vi "DisplayPanel.vi"() -> ()   [LabVIEW 2011]
uses:
  MvLVLib/MvCameraControl.lvlib
  MvLVLib/VIs/CreateGigEHandle.vi
  MvLVLib/VIs/CreateU3VHandle.vi
  <vilib>/picture/picture.llb/imagedata.ctl
panel:
  out "U3VDeviceArray":T1(array[cluster])
  out "GigEDeviceArray":T2(array[cluster])
  in  "pConvertInfo In":T3
  out "PixelFormat":u32
  out "handle out":u64
  in  "handle":u64
  in  "Rectangle":T4
  in  "image data":T5 caption="图像数据"
  out "Picture":picture
  out "PayloadSize":u32
  out "pFrameInfoEx out":T6
  out "nHeight":u32
  out "nWidth":u32
  out "Acquisision Flag":bool
  in  "Trigger Mode":bool
  in  "Continuous":bool
  out "打开标志":bool
  in  "stop":bool
  in  "Trigger Once":bool
  in  "Stop":bool
  in  "Start":bool
  in  "Open Device":bool
  in  "Close Device":bool
  in  "error in (no error) 2":errorcluster caption="错误输入（无错误）"
  in  "Refresh Devices":bool
  in  "Device List":u16(ring)
  # "Initialize"
  # "Acquisition"
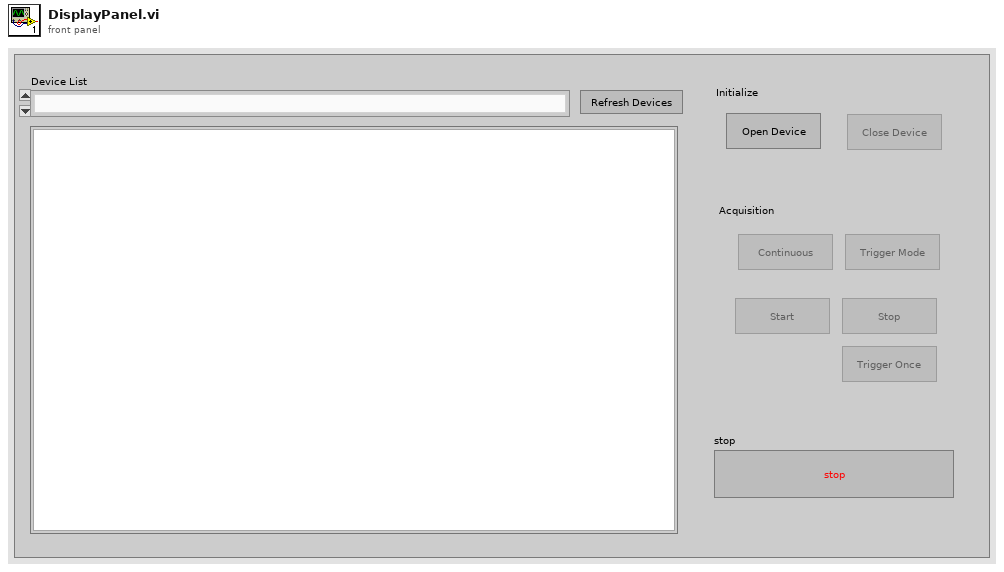
[diagram p1: front panel]
types:
  T1 = cluster{"nMajorVer":u16, "nMinorVer":u16, "nMacAddrHigh":u32, "nMacAddrLow":u32, "nTLayerType":u32, "nReserved0":u32, "nReserved1":u32, "nReserved2":u32, "nReserved3":u32, "CrtlInEndPoint":u8, "CrtlOutEndPoint":u8, "StreamEndPoint":u8, "EventEndPoint":u8, "idVendor":u16, "idProduct":u16, "nDeviceNumber":u32, "nRes0":u32, "nRes1":u32, "chDeviceGUID":string, "chVendorName":string, "chModelName":string, "chFamilyName":string, "chDeviceVersion":string, "chManufacturerName":string, "chSerialNumber":string, "chUserDefinedName":string, "nbcdUSB":u32, "nRes2":u32, "nRes3":u32}[]
  T2 = cluster{"nMajorVer":u16, "nMinorVer":u16, "nMacAddrHigh":u32, "nMacAddrLow":u32, "nTLayerType":u32, "nReserved0":u32, "nReserved1":u32, "nReserved2":u32, "nReserved3":u32, "nIpCfgOption":u32, "nIpCfgCurrent":u32, "nCurrentIp":u32, "nCurrentSubNetMask":u32, "nDefaultGateWay":u32, "chManualfacturerName":string, "chModelName":string, "chDeviceVersion":string, "chManufacturerSpecificInfo":string, "chSerialNumber":string, "chUserDefinedName":string, "nRes0":string, "nRes1":string, "nNetExport":u32, "nRes2":u32, "nRes3":u32}[]
  T3 = cluster{"nWidth":u16, "nHeight":u16, "enSrcPixelType":u32, "nSrcDataLen":u32, "enDstPixelType":u32, "nDstLen":u32, "nDstBufferSize":u32, "nRes0":u32, "nRes1":u32, "nRes2":u32, "nRes3":u32}
  T4 = cluster{"left":i16, "top":i16, "right":i16, "bottom":i16}
  T5 = typedef "imagedata.ctl" = cluster{"image type":i32, "image depth":i32, "image":u8[], "mask":u8[], "colors":u32[], "Rectangle":cluster{"left":i16, "top":i16, "right":i16, "bottom":i16}}
  T6 = cluster{"nWidth":u16, "nHeight":u16, "enPixelType":i32, "nFrameNum":u32, "nDevTimeStampHigh":u32, "nDevTimeStampLow":u32, "nReserved0":u32, "nHostTimeStamp":i64, "nFrameLen":u32, "nSecondCount]":u32, "nCycleCount":u32, "nCycleOffset":u32, "fGain":u32, "fExposureTime":u32, "nAverageBrightness":u32, "nRed":u32, "nGreen":u32, "nBlue":u32, "nFrameCounter":u32, "nTriggerIndex":u32, "nInput":u32, "nOutput":u32, "nOffsetX":u32, "nOffsetY":u32, "nReserved[0]":u32, "nReserved[1]":u32, "nReserved[2]":u32, "nReserved[3]":u32, "nReserved[4]":u32, "nReserved[5]":u32, "nReserved[6]":u32, "nReserved[7]":u32, "nReserved[8]":u32, "nReserved[9]":u32, "nReserved[10]":u32, "nReserved[11]":u32, "nReserved[12]":u32, "nReserved[13]":u32, "nReserved[14] 10":u32, "nReserved[15] 11":u32, "nReserved[16] 12":u32, "nReserved[17] 13":u32, "nReserved[18] 14":u32, "nReserved[19] 15":u32, "nReserved[20] 16":u32, "nReserved[21] 17":u32, "nReserved[22] 18":u32, "nReserved[23] 19":u32, "nReserved[24] 20":u32, "nReserved[25] 21":u32, "nReserved[26] 22":u32, "nReserved[27] 23":u32, "nReserved[28] 24":u32, "nReserved[29] 25":u32, "nReserved[30] 26":u32, "nReserved[31] 27":u32, "nReserved[32] 28":u32, "nReserved[33] 29":u32, "nReserved[34] 30":u32, "nReserved[35] 31":u32, "nReserved[36] 32":u32, "nReserved[37] 33":u32, "nReserved[38] 34":u32, "nReserved[39] 35":u32, "nReserved[40] 36":u32}
  T7 = enum8{"Enabled", "Disabled", "Disabled and Grayed Out"}
  T8 = cluster{"nCurValue":u32, "nMax":u32, "nMin":u32, "nInc":u32, "nReserved[0]":u32, "nReserved[1]":u32, "nReserved[2]":u32, "nReserved[3]":u32}
  T9 = cluster{"nCurValue":u32, "nSupportedNum":u32, "nSupportValue[0]":u32, "nSupportValue[1]":u32, "nSupportValue[2]":u32, "nSupportValue[3]":u32, "nSupportValue[4]":u32, "nSupportValue[5]":u32, "nSupportValue[6]":u32, "nSupportValue[7]":u32, "nSupportValue[8]":u32, "nSupportValue[9]":u32, "nSupportValue[10]":u32, "nSupportValue[11]":u32, "nSupportValue[12]":u32, "nSupportValue[13]":u32, "nSupportValue[14]":u32, "nSupportValue[15]":u32, "nSupportValue[16]":u32, "nSupportValue[17]":u32, "nSupportValue[18]":u32, "nSupportValue[19]":u32, "nSupportValue[20]":u32, "nSupportValue[21]":u32, "nSupportValue[22]":u32, "nSupportValue[23]":u32, "nSupportValue[24]":u32, "nSupportValue[25]":u32, "nSupportValue[26]":u32, "nSupportValue[27]":u32, "nSupportValue[28]":u32, "nSupportValue[29]":u32, "nSupportValue[30]":u32, "nSupportValue[31]":u32, "nSupportValue[32]":u32, "nSupportValue[33]":u32, "nSupportValue[34]":u32, "nSupportValue[35]":u32, "nSupportValue[36]":u32, "nSupportValue[37]":u32, "nSupportValue[38]":u32, "nSupportValue[39]":u32, "nSupportValue[40]":u32, "nSupportValue[41]":u32, "nSupportValue[42]":u32, "nSupportValue[43]":u32, "nSupportValue[44]":u32, "nSupportValue[45]":u32, "nSupportValue[46]":u32, "nSupportValue[47]":u32, "nSupportValue[48]":u32, "nSupportValue[49]":u32, "nSupportValue[50]":u32, "nSupportValue[51]":u32, "nSupportValue[52]":u32, "nSupportValue[53]":u32, "nSupportValue[54]":u32, "nSupportValue[55]":u32, "nSupportValue[56]":u32, "nSupportValue[57]":u32, "nSupportValue[58]":u32, "nSupportValue[59]":u32, "nSupportValue[60]":u32, "nSupportValue[61]":u32, "nSupportValue[62]":u32, "nSupportValue[63]":u32, "nReserved[0]":u32, "nReserved[1]":u32, "nReserved[2]":u32, "nReserved[3]":u32}
  T10 = cluster{"nMajorVer":u16, "nMinorVer":u16, "nMacAddrHigh":u32, "nMacAddrLow":u32, "nTLayerType":u32, "nReserved0":u32, "nReserved1":u32, "nReserved2":u32, "nReserved3":u32, "CrtlInEndPoint":u8, "CrtlOutEndPoint":u8, "StreamEndPoint":u8, "EventEndPoint":u8, "idVendor":u16, "idProduct":u16, "nDeviceNumber":u32, "nRes0":u32, "nRes1":u32, "chDeviceGUID":string, "chVendorName":string, "chModelName":string, "chFamilyName":string, "chDeviceVersion":string, "chManufacturerName":string, "chSerialNumber":string, "chUserDefinedName":string, "nbcdUSB":u32, "nRes2":u32, "nRes3":u32}
  T11 = cluster{"nMajorVer":u16, "nMinorVer":u16, "nMacAddrHigh":u32, "nMacAddrLow":u32, "nTLayerType":u32, "nReserved0":u32, "nReserved1":u32, "nReserved2":u32, "nReserved3":u32, "nIpCfgOption":u32, "nIpCfgCurrent":u32, "nCurrentIp":u32, "nCurrentSubNetMask":u32, "nDefaultGateWay":u32, "chManualfacturerName":string, "chModelName":string, "chDeviceVersion":string, "chManufacturerSpecificInfo":string, "chSerialNumber":string, "chUserDefinedName":string, "nRes0":string, "nRes1":string, "nNetExport":u32, "nRes2":u32, "nRes3":u32}
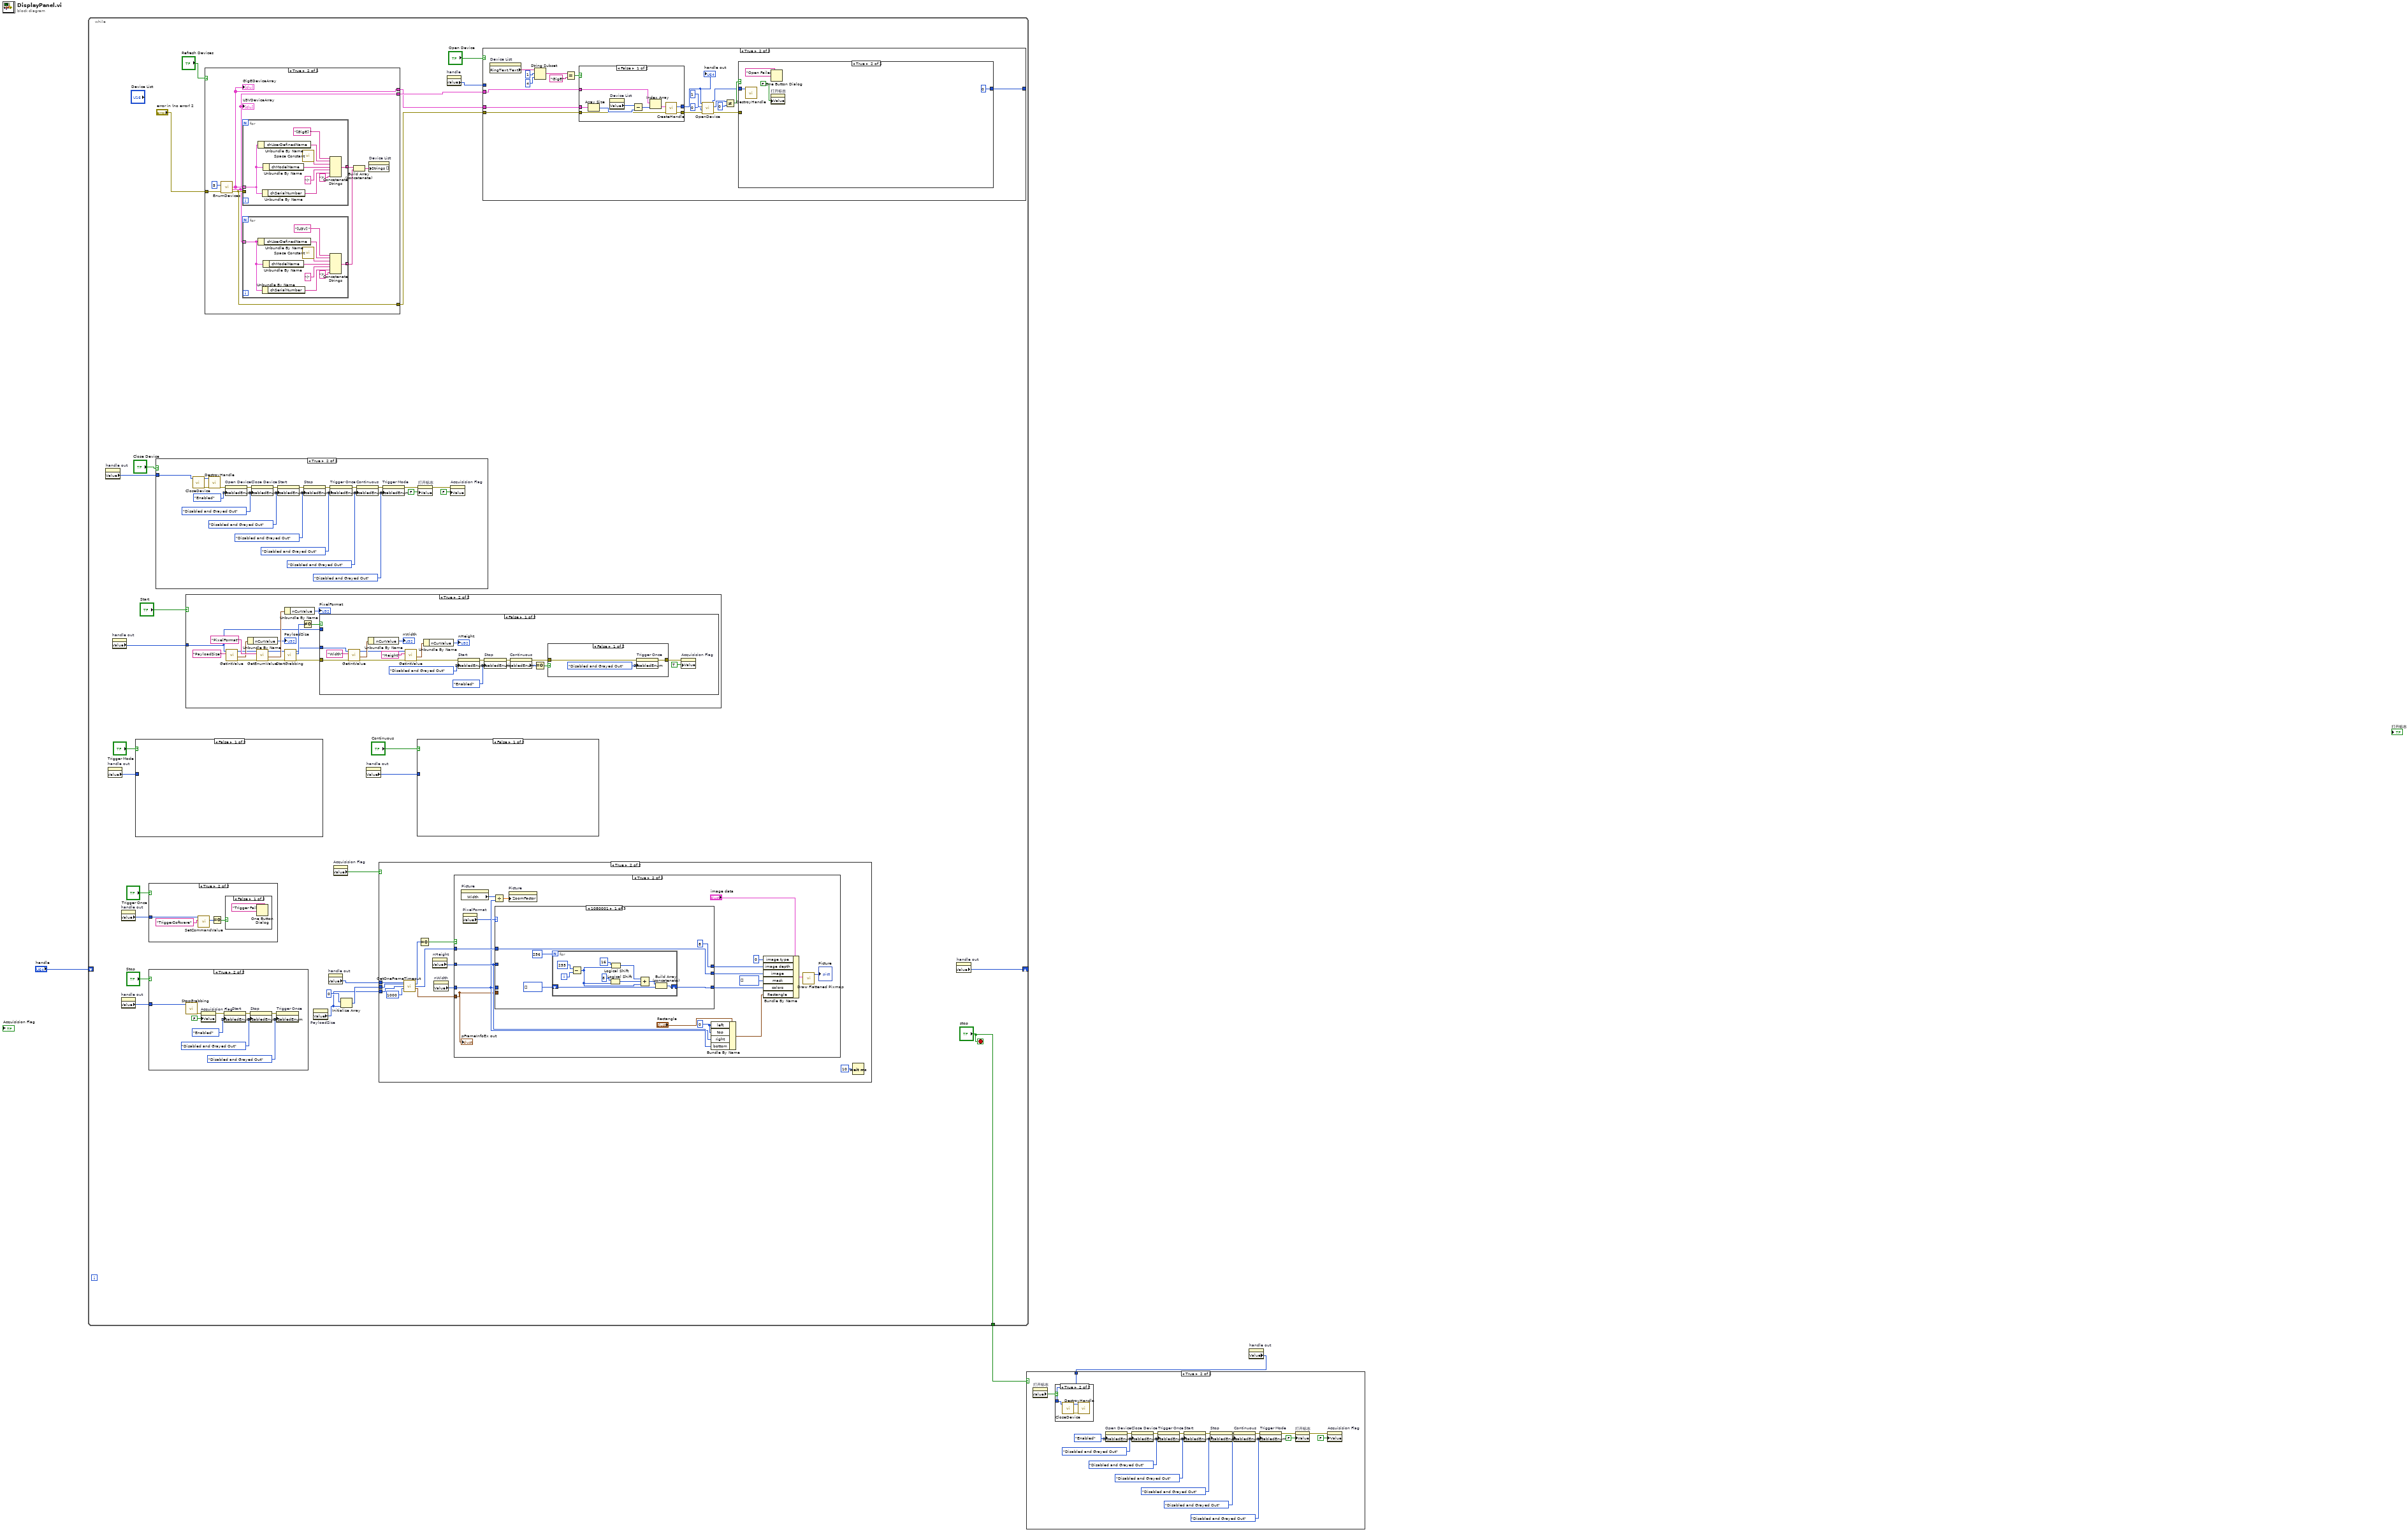
[diagram p0: block diagram]
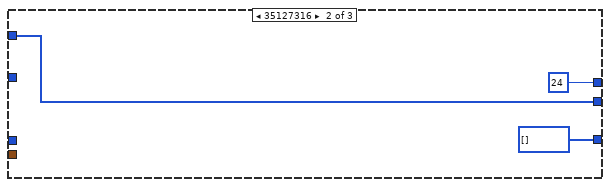
[diagram p6: hidden frame]
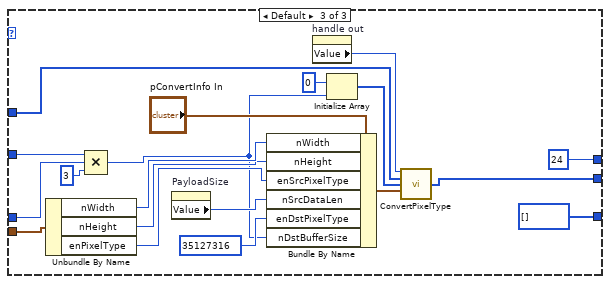
[diagram p7: hidden frame]
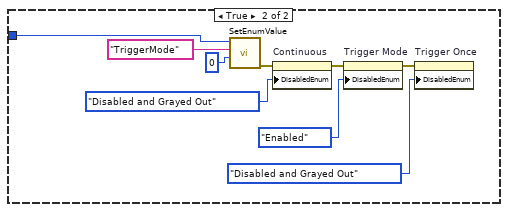
[diagram p9: hidden frame]
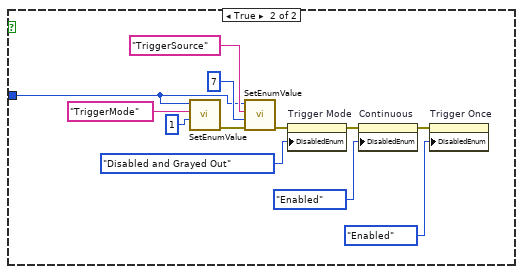
[diagram p10: hidden frame]
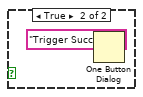
[diagram p12: hidden frame]
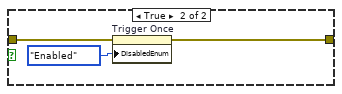
[diagram p14: hidden frame]
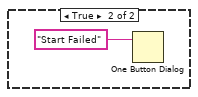
[diagram p15: hidden frame]
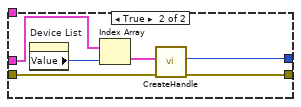
[diagram p18: hidden frame]
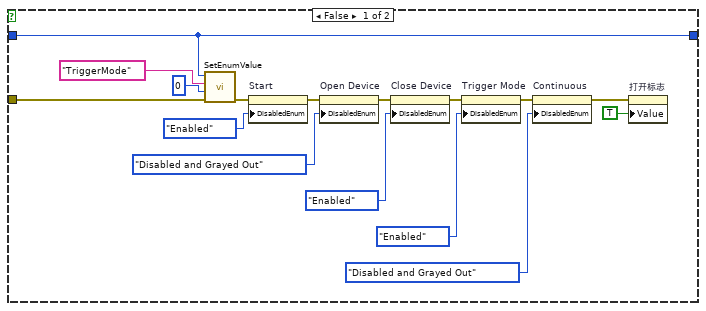
[diagram p19: hidden frame]
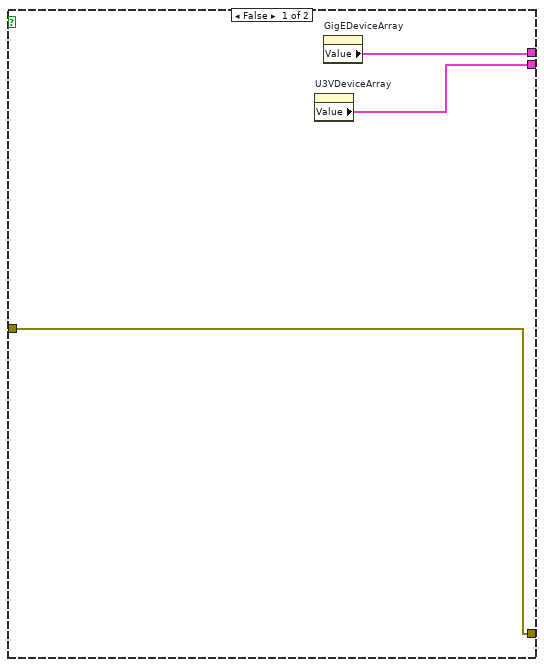
[diagram p20: hidden frame]
diagram:
  n1 = while {
    tunnel: ["stop"] -> w3
    shift-right: [w17] -> _
    shift-left: "handle" -> [_]
    stop <- "stop" stop-if-true
    n2 = property on="handle out" class="DigNum (strict)"() -> ("Value"=w15:u64)  [unwired: 2 in, 2 out]
    n3 = property on="handle out" class="DigNum (strict)"() -> ("Value"=w10:u64)  [unwired: 2 in, 2 out]
    n4 = property on="handle out" class="DigNum (strict)"() -> ("Value"=w11:u64)  [unwired: 2 in, 2 out]
    n5 = property on="handle out" class="DigNum (strict)"() -> ("Value"=w14:u64)  [unwired: 2 in, 2 out]
    n6 = property on="handle out" class="DigNum (strict)"() -> ("Value"=w13:u64)  [unwired: 2 in, 2 out]
    n7 = case shown="False" "Trigger Mode" {
      tunnel: w10 -> [_ w114]
      frame False {
      }
      frame True {
        n8 = call "SetEnumValue.vi"("nValue"=u32 1, "strKey"="TriggerMode", "handle"=w114) -> ("error out"=w120:errorcluster)  [unwired: 6 in, 2 out]
        n9 = call "SetEnumValue.vi"("error in (no error)"=w120, "nValue"=u32 7, "strKey"="TriggerSource", "handle"=w114) -> ("error out"=w119:errorcluster)  [unwired: 5 in, 2 out]
        n10 = property on="Trigger Mode" class="Bool"(error in=w119, "DisabledEnum"=T7."Disabled and Grayed Out" ("禁用")) -> (error out=w118:errorcluster)  [unwired: 1 in, 1 out]
        n11 = property on="Continuous" class="Bool"(error in=w118, "DisabledEnum"=T7."Enabled" ("禁用")) -> (error out=w116:errorcluster)  [unwired: 1 in, 1 out]
        n12 = property on="Trigger Once" class="Bool"(error in=w116, "DisabledEnum"=T7."Enabled" ("禁用")) -> ()  [unwired: 1 in, 2 out]
      }
    }
    n13 = case shown="True" "Trigger Once" {
      tunnel: w14 -> [_ w129]
      frame False {
      }
      frame True {
        n14 = call "SetCommandValue.vi"("strValue"="TriggerSoftware", "handle"=w129) -> ("function return"=w127:i32)  [unwired: 7 in, 2 out]
        n15 = Equal To 0?(x=w127) -> (x = 0?=w126:bool)
        n16 = case shown="False" w126 {
          frame False {
            n17 = One Button Dialog(message="Trigger Failed") -> ()  [unwired: 1 in, 1 out]
          }
          frame True {
            n18 = One Button Dialog(message="Trigger Success") -> ()  [unwired: 1 in, 1 out]
          }
        }
      }
    }
    n19 = case shown="True" "Stop" {
      tunnel: w13 -> [_ w104]
      frame False {
      }
      frame True {
        n20 = call "StopGrabbing.vi"("handle"=w104) -> ("error out"=w103:errorcluster)  [unwired: 8 in, 2 out]
        n21 = property on="Acquisision Flag" class="Bool (strict)"(error in=w103, "Value"=FALSE ("采集标志")) -> (error out=w98:errorcluster)  [unwired: 1 in, 1 out]
        n22 = property on="Start" class="Bool"(error in=w98, "DisabledEnum"=T7."Enabled" ("禁用")) -> (error out=w97:errorcluster)  [unwired: 1 in, 1 out]
        n23 = property on="Stop" class="Bool"(error in=w97, "DisabledEnum"=T7."Disabled and Grayed Out" ("禁用")) -> (error out=w96:errorcluster)  [unwired: 1 in, 1 out]
        n24 = property on="Trigger Once" class="Bool"(error in=w96, "DisabledEnum"=T7."Disabled and Grayed Out" ("禁用")) -> ()  [unwired: 1 in, 2 out]
      }
    }
    n25 = case shown="True" "Close Device" {
      tunnel: w15 -> [_ w175]
      frame False {
      }
      frame True {
        n26 = call "CloseDevice.vi"("handle"=w175) -> ("error out"=w177:errorcluster, "handle out"=w174:u64)  [unwired: 8 in, 1 out]
        n27 = call "DestroyHandle.vi"("error in (no error)"=w177, "handle"=w174) -> ("error out"=w176:errorcluster)  [unwired: 8 in, 1 out]
        n28 = property on="Open Device" class="Bool"(error in=w176, "DisabledEnum"=T7."Enabled" ("禁用")) -> (error out=w190:errorcluster)  [unwired: 1 in, 1 out]
        n29 = property on="Close Device" class="Bool"(error in=w190, "DisabledEnum"=T7."Disabled and Grayed Out" ("禁用")) -> (error out=w189:errorcluster)  [unwired: 1 in, 1 out]
        n30 = property on="Start" class="Bool"(error in=w189, "DisabledEnum"=T7."Disabled and Grayed Out" ("禁用")) -> (error out=w188:errorcluster)  [unwired: 1 in, 1 out]
        n31 = property on="Stop" class="Bool"(error in=w188, "DisabledEnum"=T7."Disabled and Grayed Out" ("禁用")) -> (error out=w187:errorcluster)  [unwired: 1 in, 1 out]
        n32 = property on="Trigger Once" class="Bool"(error in=w187, "DisabledEnum"=T7."Disabled and Grayed Out" ("禁用")) -> (error out=w184:errorcluster)  [unwired: 1 in, 1 out]
        n33 = property on="Continuous" class="Bool"(error in=w184, "DisabledEnum"=T7."Disabled and Grayed Out" ("禁用")) -> (error out=w182:errorcluster)  [unwired: 1 in, 1 out]
        n34 = property on="Trigger Mode" class="Bool"(error in=w182, "DisabledEnum"=T7."Disabled and Grayed Out" ("禁用")) -> (error out=w181:errorcluster)  [unwired: 1 in, 1 out]
        n35 = property on="打开标志" class="Bool (strict)"(error in=w181, "Value"=FALSE ("打开标志")) -> (error out=w179:errorcluster)  [unwired: 1 in, 1 out]
        n36 = property on="Acquisision Flag" class="Bool (strict)"(error in=w179, "Value"=FALSE ("采集标志")) -> ()  [unwired: 1 in, 2 out]
      }
    }
    n37 = case shown="True" "Start" {
      tunnel: w11 -> [_ w136]
      frame False {
      }
      frame True {
        n38 = call "GetIntValue.vi"("strKey"="PayloadSize", "handle"=w136) -> ("error out"=w142:errorcluster, "pIntValue out"=w138:T8, "handle out"=w134:u64)  [unwired: 6 in, 1 out]
        n39 = Unbundle By Name(w138) -> ("nCurValue"=→"PayloadSize":u32)
        n40 = call "GetEnumValue.vi"("error in (no error)"=w142, "strKey"="PixelFormat", "handle"=w134) -> ("error out"=w141:errorcluster, "pEnumValue out"=w143:T9, "handle out"=w133:u64)  [unwired: 5 in, 1 out]
        n41 = Unbundle By Name(w143) -> ("nCurValue"=→"PixelFormat":u32)
        n42 = call "StartGrabbing.vi"("error in (no error)"=w141, "handle"=w133) -> ("error out"=w140:errorcluster, "function return"=w146:i32, "handle out"=w132:u64)  [unwired: 7 in]
        n43 = Not Equal To 0?(x=w146) -> (x != 0?=w145:bool)
        n44 = case shown="False" w145 {
          tunnel: w136 -> [_ _]
          tunnel: w140 -> [w149 _]
          tunnel: w132 -> [w148 _]
          frame False {
            n45 = call "GetIntValue.vi"("error in (no error)"=w149, "strKey"="Width", "handle"=w148) -> ("error out"=w156:errorcluster, "pIntValue out"=w150:T8, "handle out"=w147:u64)  [unwired: 5 in, 1 out]
            n46 = Unbundle By Name(w150) -> ("nCurValue"=→"nWidth":u32)
            n47 = call "GetIntValue.vi"("error in (no error)"=w156, "strKey"="Height", "handle"=w147) -> ("error out"=w155:errorcluster, "pIntValue out"=w153:T8)  [unwired: 5 in, 2 out]
            n48 = Unbundle By Name(w153) -> ("nCurValue"=→"nHeight":u32)
            n49 = property on="Start" class="Bool"(error in=w155, "DisabledEnum"=T7."Disabled and Grayed Out" ("禁用")) -> (error out=w165:errorcluster)  [unwired: 1 in, 1 out]
            n50 = property on="Stop" class="Bool"(error in=w165, "DisabledEnum"=T7."Enabled" ("禁用")) -> (error out=w151:errorcluster)  [unwired: 1 in, 1 out]
            n51 = property on="Continuous" class="Bool"(error in=w151) -> (error out=w161:errorcluster, "DisabledEnum"=w162:T7)  [unwired: 1 in, 1 out]
            n52 = Equal To 0?(x=w162) -> (x = 0?=w163:bool)
            n53 = case shown="False" w163 {
              tunnel: w161 -> [w168 w171]
              tunnel: [w167 w170] -> w160
              frame False {
                n54 = property on="Trigger Once" class="Bool"(error in=w168, "DisabledEnum"=T7."Disabled and Grayed Out" ("禁用")) -> (error out=w167:errorcluster)  [unwired: 1 in, 1 out]
              }
              frame True {
                n55 = property on="Trigger Once" class="Bool"(error in=w171, "DisabledEnum"=T7."Enabled" ("禁用")) -> (error out=w170:errorcluster)  [unwired: 1 in, 1 out]
              }
            }
            n56 = property on="Acquisision Flag" class="Bool (strict)"(error in=w160, "Value"=TRUE ("采集标志")) -> ()  [unwired: 1 in, 2 out]
          }
          frame True {
            n57 = One Button Dialog(message="Start Failed") -> ()  [unwired: 1 in, 1 out]
          }
        }
      }
    }
    n58 = case shown="True" "Refresh Devices" {
      tunnel: [w252 w259] -> w19
      tunnel: "error in (no error) 2" -> [w252 w258]
      tunnel: [w250 w253] -> w5
      tunnel: [w251 w254] -> w4
      frame False {
        n59 = property on="U3VDeviceArray" class="Arr (strict)"() -> ("Value"=w250:T1)  [unwired: 2 in, 2 out]
        n60 = property on="GigEDeviceArray" class="Arr (strict)"() -> ("Value"=w251:T2)  [unwired: 2 in, 2 out]
      }
      frame True {
        n61 = call "EnumDevices.vi"("nLayerType"=u32 5, "error in (no error)"=w258) -> ("GigEDeviceArray"=w254:T2, "U3VDeviceArray"=w253:T1, "error out"=w259:errorcluster)  [unwired: 9 in, 2 out]
        "GigEDeviceArray" <- w254
        "U3VDeviceArray" <- w253
        n62 = for {
          tunnel: w259 -> [_]
          tunnel: w254 -> [w272] mode=indexing
          tunnel: [w271] -> w257 mode=indexing
          n63 = Unbundle By Name(w272) -> ("chUserDefinedName"=w275:string)
          n64 = Unbundle By Name(w272) -> ("chSerialNumber"=w273:string)
          n65 = Unbundle By Name(w272) -> ("chModelName"=w274:string)
          n66 = call <vilib>:"Space Constant.vi"() -> ("String"=w278:string)
          n67 = Concatenate Strings("[GigE] " ("字符串"), w275, w278, w274, "(" ("字符串"), w273, ")" ("字符串")) -> (w271:string)
        }
        n68 = for {
          tunnel: w253 -> [w265] mode=indexing
          tunnel: [w262] -> w256 mode=indexing
          n69 = Unbundle By Name(w265) -> ("chUserDefinedName"=w269:string)
          n70 = Unbundle By Name(w265) -> ("chSerialNumber"=w264:string)
          n71 = Unbundle By Name(w265) -> ("chModelName"=w267:string)
          n72 = call <vilib>:"Space Constant.vi"() -> ("String"=w268:string)
          n73 = Concatenate Strings("[U3V] " ("字符串"), w269, w268, w267, "(" ("字符串"), w264, ")" ("字符串")) -> (w262:string)
        }
        n74 = Build Array (concatenate)(w257, w256) -> (w255:string[])
        n75 = property on="Device List" class="Ring (strict)"("Strings []"=w255) -> ()  [unwired: 2 in, 2 out]
      }
    }
    n76 = property on="PayloadSize" class="DigNum (strict)"() -> ("Value"=w6:u32)  [unwired: 2 in, 2 out]
    n77 = property on="handle out" class="DigNum (strict)"() -> ("Value"=w12:u64)  [unwired: 2 in, 2 out]
    n78 = property on="Acquisision Flag" class="Bool (strict)"() -> ("Value"=w21:bool)  [unwired: 2 in, 2 out]
    n79 = Initialize Array(u8 0 ("元素"), w6) -> (w7:u8[])
    n80 = property on="handle out" class="DigNum (strict)"() -> ("Value"=w9:u64)  [unwired: 2 in, 2 out]
    n81 = case shown="True" w21 {
      tunnel: w12 -> [_ w35]
      tunnel: w7 -> [_ w34]
      tunnel: w6 -> [_ w33]
      frame False {
      }
      frame True {
        n82 = call "GetOneFrameTimeout.vi"("handle"=w35, "pData"=w34, "nDataSize"=w33, "nMsec"=1000) -> ("function return"=w32:i32, "pData Out"=w31:u8[], "pFrameInfoEx out"=w30:T6)  [unwired: 7 in, 2 out]
        n83 = Equal To 0?(x=w32) -> (x = 0?=w39:bool)
        n84 = property on="nHeight" class="DigNum (strict)"() -> ("Value"=w37:u32)  [unwired: 2 in, 2 out]
        n85 = property on="nWidth" class="DigNum (strict)"() -> ("Value"=w38:u32)  [unwired: 2 in, 2 out]
        n86 = case shown="True" w39 {
          tunnel: w31 -> [_ w48]
          tunnel: w38 -> [_ w46]
          tunnel: w37 -> [_ w47]
          tunnel: w30 -> [_ w41]
          frame False {
          }
          frame True {
            w55 = i16 0 ("left")
            n87 = property on="Picture" class="Pict"() -> ("Width"=w50:u32)  [unwired: 2 in, 2 out]
            n88 = property on="PixelFormat" class="DigNum (strict)"() -> ("Value"=w42:u32)  [unwired: 2 in, 2 out]
            n89 = Divide(x=w50, y=w46) -> (x/y=w49:dbl)
            n90 = case shown="1080001" w42 {
              tunnel: w48 -> [w61 w76 w92]
              tunnel: w47 -> [_ _ w89]
              tunnel: w46 -> [_ _ w88]
              tunnel: [w61 w76 w77] -> w45
              tunnel: [8 24 24] -> w44
              tunnel: [w59 i32[] [] i32[] []] -> w43
              tunnel: w41 -> [_ _ w78]
              frame 17301505 {
                n91 = for {
                  N: 256 -> [_]
                  shift-right: [w68] -> w59
                  shift-left: i32[] [] ("数组") -> [w67]
                  i -> [w64]
                  n92 = Subtract(x=255, y=w64) -> (x-y=w65:i32)
                  n93 = Logical Shift(y=i16 8, x=w65) -> (x << y=w70:i32)
                  n94 = Logical Shift(y=16 ("x"), x=w65) -> (x << y=w71:i32)
                  n95 = Compound Arithmetic op=ADD(w71, w70, w65) -> (w69:i32)
                  n96 = Build Array (concatenate)(w69, w67) -> (w68:i32[])
                }
              }
              frame 35127316 {
              }
              frame Default {
                n97 = Unbundle By Name(w78) -> ("nWidth"=w87:u16, "nHeight"=w86:u16, "enPixelType"=w85:i32)
                n98 = Compound Arithmetic op=MULTIPLY(w89, w88, u32 3 ("值")) -> (w82:u32)
                n99 = property on="PayloadSize" class="DigNum (strict)"() -> ("Value"=w84:u32)  [unwired: 2 in, 2 out]
                n100 = Bundle By Name(cluster="pConvertInfo In", "nWidth"=w87, "nHeight"=w86, "enSrcPixelType"=w85, "nSrcDataLen"=w84, "enDstPixelType"=u32 35127316, "nDstBufferSize"=w82) -> (w81:T3)
                n101 = property on="handle out" class="DigNum (strict)"() -> ("Value"=w93:u64)  [unwired: 2 in, 2 out]
                n102 = Initialize Array(u8 0 ("元素"), w82) -> (w91:u8[])
                n103 = call "ConvertPixelType.vi"("handle"=w93, "pSrcData"=w92, "pDstBuf In"=w91, "pConvertInfo In"=w81) -> ("pDstBuf Out"=w77:u8[])  [unwired: 7 in, 4 out]
              }
            }
            n104 = property on="Picture" class="Pict"("ZoomFactor"=w49) -> ()  [unwired: 2 in, 2 out]
            n105 = Bundle By Name(cluster="Rectangle", "left"=w55, "top"=w55, "right"=w46, "bottom"=w47) -> (w52:T4)
            n106 = Bundle By Name(cluster="image data", "image type"=0, "image depth"=w44, "image"=w45, "mask"=u8[] [], "colors"=w43, "Rectangle"=w52) -> (w51:T5)
            n107 = call <vilib>:"Draw Flattened Pixmap.vi"("image data"=w51) -> ("new picture"=→"Picture":picture)  [unwired: 8 in]
            "pFrameInfoEx out" <- w41
          }
        }
        n108 = Wait (ms)(milliseconds to wait=u32 10 ("等待时间（毫秒）")) -> ()  [unwired: 1 out]
      }
    }
    n109 = case shown="False" "Continuous" {
      tunnel: w9 -> [_ w105]
      frame False {
      }
      frame True {
        n110 = call "SetEnumValue.vi"("nValue"=u32 0, "strKey"="TriggerMode", "handle"=w105) -> ("error out"=w106:errorcluster)  [unwired: 6 in, 2 out]
        n111 = property on="Continuous" class="Bool"(error in=w106, "DisabledEnum"=T7."Disabled and Grayed Out" ("禁用")) -> (error out=w110:errorcluster)  [unwired: 1 in, 1 out]
        n112 = property on="Trigger Mode" class="Bool"(error in=w110, "DisabledEnum"=T7."Enabled" ("禁用")) -> (error out=w108:errorcluster)  [unwired: 1 in, 1 out]
        n113 = property on="Trigger Once" class="Bool"(error in=w108, "DisabledEnum"=T7."Disabled and Grayed Out" ("禁用")) -> ()  [unwired: 1 in, 2 out]
      }
    }
    n114 = property on="handle" class="DigNum (strict)"() -> ("Value"=w16:u64)  [unwired: 2 in, 2 out]
    n115 = case shown="True" "Open Device" {
      tunnel: [w195 w207] -> _
      tunnel: w16 -> [w195 _]
      tunnel: w19 -> [_ w206]
      tunnel: w5 -> [_ w197]
      tunnel: w4 -> [_ w196]
      frame False {
      }
      frame True {
        n116 = property on="Device List" class="Ring (strict)"() -> ("RingText.Text"=w205:string)  [unwired: 2 in, 2 out]
        n117 = String Subset(string=w205, offset (0)=1 ("偏移量(0)"), length (rest)=4 ("长度（剩余）")) -> (substring=w202:string)
        n118 = Equal?(x=w202, y="GigE") -> (x = y?=w201:bool)
        n119 = case shown="False" w201 {
          tunnel: [w217 w226] -> w212
          tunnel: [w216 w225] -> w208
          tunnel: w196 -> [w221 w228]
          tunnel: w206 -> [w218 w227]
          tunnel: w197 -> [w223 _]
          frame False {
            n120 = Array Size(array=w221) -> (size(s)=w220:i32)
            n121 = property on="Device List" class="Ring (strict)"() -> ("Value"=w222:u16)  [unwired: 2 in, 2 out]
            n122 = Subtract(x=w222, y=w220) -> (x-y=w219:i32)
            n123 = Index Array(array=w223, index=w219) -> (element=w215:T10)
            n124 = call-poly "CreateHandle.vi"("error in (no error)"=w218, "U3VDevice"=w215) -> ("error out"=w217:errorcluster, "handle"=w216:u64)  [unwired: 6 in, 1 out]
          }
          frame True {
            n125 = property on="Device List" class="Ring (strict)"() -> ("Value"=w229:u16)  [unwired: 2 in, 2 out]
            n126 = Index Array(array=w228, index=w229) -> (element=w224:T11)
            n127 = call-poly "CreateHandle.vi"("error in (no error)"=w227, "GigEDevice"=w224) -> ("error out"=w226:errorcluster, "handle"=w225:u64)  [unwired: 6 in, 1 out]
          }
        }
        "handle out" <- w208
        n128 = call "OpenDevice.vi"("error in (no error)"=w212, "nSwitchoverKey"=u16 0, "nAccessMode"=u32 1, "handle"=w208) -> ("error out"=w209:errorcluster, "return"=w199:i32, "handle out"=w198:u64)  [unwired: 5 in]
        n129 = Not Equal?(x=w199, y=0) -> (x != y?=w213:bool)
        n130 = case shown="True" w213 {
          tunnel: w198 -> [w230 w247]
          tunnel: w209 -> [w231 _]
          tunnel: [w230 u64 0 ("handle")] -> w207
          frame False {
            n131 = call "SetEnumValue.vi"("error in (no error)"=w231, "nValue"=u32 0, "strKey"="TriggerMode", "handle"=w230) -> ("error out"=w242:errorcluster)  [unwired: 5 in, 2 out]
            n132 = property on="Start" class="Bool"(error in=w242, "DisabledEnum"=T7."Enabled" ("禁用")) -> (error out=w240:errorcluster)  [unwired: 1 in, 1 out]
            n133 = property on="Open Device" class="Bool"(error in=w240, "DisabledEnum"=T7."Disabled and Grayed Out" ("禁用")) -> (error out=w239:errorcluster)  [unwired: 1 in, 1 out]
            n134 = property on="Close Device" class="Bool"(error in=w239, "DisabledEnum"=T7."Enabled" ("禁用")) -> (error out=w236:errorcluster)  [unwired: 1 in, 1 out]
            n135 = property on="Trigger Mode" class="Bool"(error in=w236, "DisabledEnum"=T7."Enabled" ("禁用")) -> (error out=w234:errorcluster)  [unwired: 1 in, 1 out]
            n136 = property on="Continuous" class="Bool"(error in=w234, "DisabledEnum"=T7."Disabled and Grayed Out" ("禁用")) -> (error out=w232:errorcluster)  [unwired: 1 in, 1 out]
            n137 = property on="打开标志" class="Bool (strict)"(error in=w232, "Value"=TRUE ("布尔")) -> ()  [unwired: 1 in, 2 out]
          }
          frame True {
            n138 = call "DestroyHandle.vi"("handle"=w247) -> ()  [unwired: 9 in, 2 out]
            n139 = One Button Dialog(message="Open Failed") -> ()  [unwired: 1 in, 1 out]
            n140 = property on="打开标志" class="Bool (strict)"("Value"=FALSE) -> ()  [unwired: 2 in, 2 out]
          }
        }
      }
    }
    n141 = property on="handle out" class="DigNum (strict)"() -> ("Value"=w17:u64)  [unwired: 2 in, 2 out]
  }
  n142 = property on="handle out" class="DigNum (strict)"() -> ("Value"=w1:u64)  [unwired: 2 in, 2 out]
  n143 = case shown="True" w3 {
    tunnel: w1 -> [_ w292]
    frame False {
    }
    frame True {
      n144 = property on="打开标志" class="Bool (strict)"() -> ("Value"=w283:bool)  [unwired: 2 in, 2 out]
      n145 = case shown="True" w283 {
        tunnel: w292 -> [_ w299]
        frame False {
        }
        frame True {
          n146 = call "CloseDevice.vi"("handle"=w299) -> ("error out"=w300:errorcluster, "handle out"=w298:u64)  [unwired: 8 in, 1 out]
          n147 = call "DestroyHandle.vi"("error in (no error)"=w300, "handle"=w298) -> ()  [unwired: 8 in, 2 out]
        }
      }
      n148 = property on="Open Device" class="Bool"("DisabledEnum"=T7."Enabled" ("禁用")) -> (error out=w291:errorcluster)  [unwired: 2 in, 1 out]
      n149 = property on="Close Device" class="Bool"(error in=w291, "DisabledEnum"=T7."Disabled and Grayed Out" ("禁用")) -> (error out=w290:errorcluster)  [unwired: 1 in, 1 out]
      n150 = property on="Trigger Once" class="Bool"(error in=w290, "DisabledEnum"=T7."Disabled and Grayed Out" ("禁用")) -> (error out=w289:errorcluster)  [unwired: 1 in, 1 out]
      n151 = property on="Start" class="Bool"(error in=w289, "DisabledEnum"=T7."Disabled and Grayed Out" ("禁用")) -> (error out=w288:errorcluster)  [unwired: 1 in, 1 out]
      n152 = property on="Stop" class="Bool"(error in=w288, "DisabledEnum"=T7."Disabled and Grayed Out" ("禁用")) -> (error out=w287:errorcluster)  [unwired: 1 in, 1 out]
      n153 = property on="Continuous" class="Bool"(error in=w287, "DisabledEnum"=T7."Disabled and Grayed Out" ("禁用")) -> (error out=w285:errorcluster)  [unwired: 1 in, 1 out]
      n154 = property on="Trigger Mode" class="Bool"(error in=w285, "DisabledEnum"=T7."Disabled and Grayed Out" ("禁用")) -> (error out=w280:errorcluster)  [unwired: 1 in, 1 out]
      n155 = property on="打开标志" class="Bool (strict)"(error in=w280, "Value"=FALSE ("打开标志")) -> (error out=w279:errorcluster)  [unwired: 1 in, 1 out]
      n156 = property on="Acquisision Flag" class="Bool (strict)"(error in=w279, "Value"=FALSE ("采集标志")) -> ()  [unwired: 1 in, 2 out]
    }
  }
